vi "Create NI 9475 - Counter Driven Output.vi"(8 "error in":errorcluster, 10 "drive from slot":T1, 11 "channel settings":T2[](array[typedef])) -> (0 "error out":errorcluster, 3 "NI 9475 out":refnum<class "NI 9475.lvclass">)   [LabVIEW 2020, in "Scan Engine Scripting.lvlib" / "NI 9475.lvclass"]
doc: "Creates and configures an instance of a NI-9475 counter driven output module that can be used to set a slot in a Scan Engine custom device chassis."
uses:
  NI 9475.lvclass
  Mode Classes/Controls/counter driven output channel settings.ctl
  Channel Classes/Counter Driven Output Channel/Counter Driven State.ctl
  Mode Classes/Counter Driven Output Mode/Drive from Slot.ctl
  Mode Classes/Counter Driven Output Mode/Counter Driven Output Mode.lvclass
  C:/jenkins/workspace/ercat-custom-device_release_20.4/Custom Device Source/Scripting/Modules/Mode Classes/Mode/Mode.lvclass
  2e1475cf-b729-4d54-b40b-61f7c6ab14ce.vi
  Channel Classes/Counter Driven Output Channel/Counter Driven Output Channel.lvclass
  Scan Engine Scripting.lvlib
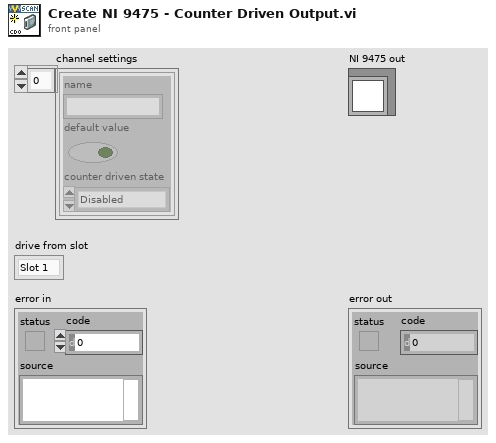
[diagram p1: front panel]
types:
  T1 = typedef "Scan Engine Scripting.lvlib/Counter Driven Output Mode.lvclass/Drive from Slot.ctl" = enum16{"Slot 1", "Slot 2", "Slot 3", "Slot 4", "Slot 5", "Slot 6", "Slot 7", "Slot 8"}
  T2 = typedef "Scan Engine Scripting.lvlib/counter driven output channel settings.ctl" = cluster{"name":string, "default value":bool, "counter driven state":T3}
  T3 = typedef "Scan Engine Scripting.lvlib/Counter Driven Output Channel.lvclass/Counter Driven State.ctl" = enum16{"Disabled", "Enabled"}
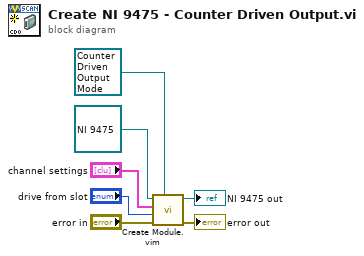
[diagram p0: block diagram]
diagram:
  n1 = call "Create Module.vim"("mode"=refnum<class "Counter Driven Output Mode.lvclass"> refnum ("Scan Engine Scripting.lvlib:Counter Driven Output Mode.lvclass"), "error in"="error in", "mode settings"="drive from slot", "channel settings"="channel settings", "module in"=refnum<class "NI 9475.lvclass"> refnum ("NI 9475 in")) -> ("error out"=→"error out":errorcluster, "module out"=→"NI 9475 out":refnum<class "NI 9475.lvclass">)  [unwired: 5 in]
